vi "Protocol Read.vi"(8 "error in":errorcluster, 9 "timeout":i32=10000, 10 "Bytes to Read":i32, 11 "protocol layer in":refnum<class "TCP Slave.lvclass">) -> (0 "error out":errorcluster, 1 "Timed out":bool, 2 "data":u8[](array[numeric]), 3 "protocol layer out":refnum<class "TCP Slave.lvclass">)   [LabVIEW 2013, in "Modbus Library - Advance.lvlib" / "TCP Slave.lvclass"]
doc: "Reads from the established TCP connection stored in the class."
uses:
  TCP Slave.lvclass
  TCP Slave.lvclass/TCP Slave.ctl
  <vilib>/Utility/error.llb/Clear Errors.vi
  TCP Shared Components/TCP Shared Components.lvlib
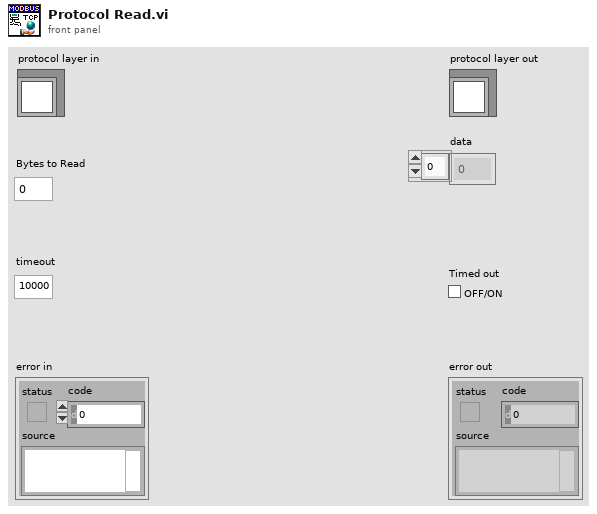
[diagram p1: front panel]
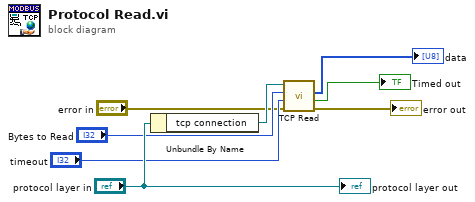
[diagram p0: block diagram]
diagram:
  n1 = Unbundle By Name("protocol layer in") -> ("tcp connection"=w7:refnum<k5>)
  n2 = call "TCP Read.vi"("error in"="error in", "timeout"="timeout", "bytes to read"="Bytes to Read", "connection ID"=w7) -> ("error out"=→"error out":errorcluster, "timed out?"=→"Timed out":bool, "data"=→"data":u8[])  [unwired: 5 in]
  "protocol layer out" <- "protocol layer in"
